vi "Untitled 1.vi"() -> ()   [LabVIEW 2018]
panel:
  in  "Path":path=path "E:/17 - Samazama na Omoi (online-audio-converter.com).wav"
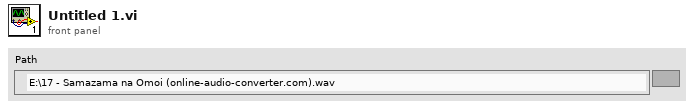
[diagram p1: front panel]
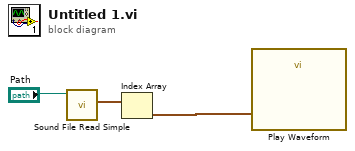
[diagram p0: block diagram]
diagram:
  n1 = call <vilib>:"Sound File Read Simple.vi"("path"="Path") -> ("data"=w2:waveform(dbl)[])  [unwired: 7 in, 3 out]
  n2 = Index Array(array=w2) -> (element=w1:waveform(dbl))  [unwired: 1 in]
  n3 = call "Play Waveform"("Data"=w1) -> ()  [unwired: 18 in, 1 out]
